vi "Transform And Project.vi"(11 "Scene in":refnum<class "Scene.lvclass">) -> (3 "Scene out":refnum<class "Scene.lvclass">)   [LabVIEW 2022 SP3, in "Application.lvlib" / "Scene.lvclass"]
uses:
  Scene.lvclass
  Libraries/3D/Vector 3D.ctl
  Scene.lvclass/Scene.ctl
  196e4586-e654-41ec-a3a4-43fea5068e8e.vi
  a59a4b44-279f-4314-be75-e28f6a03f0ec.vi
  <vilib>/Utility/High Resolution Relative Seconds.vi
  Libraries/3D/Normalise Vector.vi
  Libraries/3D/Multiply Vector By Matrix.vi
  Libraries/3D/Scale Point 3D (SGL) To Screen.vi
  Libraries/3D/Calculate Triangle Illumination.vi
  <vilib>/Utility/colorconv.llb/Color to RGB.vi
  Libraries/3D/Dot Product.vi
  <vilib>/Utility/colorconv.llb/RGB to Color.vi
  <userlib>/_OpenG.lib/array/array.llb/Sort Array__ogtk.vi
  <userlib>/_OpenG.lib/array/array.llb/Sort 1D Array (SGL)__ogtk.vi
  Libraries/3D/3D.lvlib
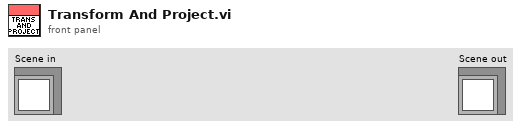
[diagram p1: front panel]
types:
  T1 = typedef "3D.lvlib/Vector 3D.ctl" = cluster{"x":sgl, "y":sgl, "z":sgl}
  T2 = typedef "3D.lvlib/Object.ctl" = cluster{"Triangles":T3[], "Diffuse Colour":u32, "Transform":T4}
  T3 = typedef "3D.lvlib/Triangle 3D.ctl" = cluster{"Point 1":T1, "Point 2":T1, "Point 3":T1}
  T4 = typedef "3D.lvlib/Transform.ctl" = cluster{"Position":T1, "Rotation":T1, "Scale":T1}
  T5 = typedef "Raster.lvlib/Screen Dimensions.ctl" = cluster{"Width":u32, "Height":u32}
  T6 = typedef "3D.lvlib/Triangle 3D With Colour.ctl" = cluster{"Point 1":T1, "Point 2":T1, "Point 3":T1, "Fill Colour":u32}
  T7 = typedef "3D.lvlib/Triangle 2D.ctl" = cluster{"Point 1":T8, "Point 2":T8, "Point 3":T8, "Fill Colour":u32}
  T8 = typedef "3D.lvlib/Point 2D.ctl" = cluster{"x":sgl, "y":sgl}
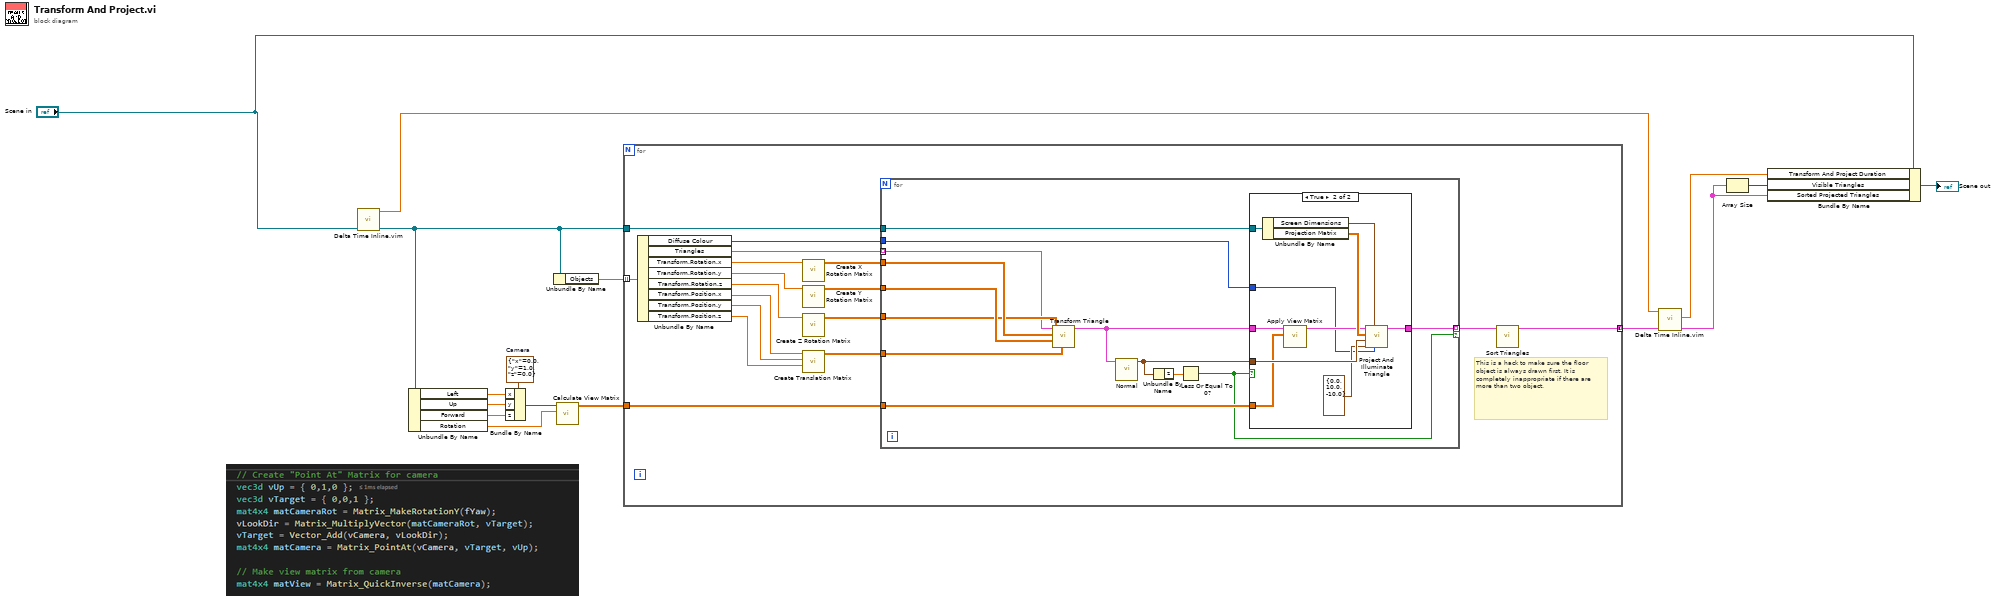
[diagram p0: block diagram]
diagram:
  w14 = T1 {"x"=0.0, "y"=1.0, "z"=0.0}  # Camera
  n1 = call "Delta Time Inline.vim"("value in"="Scene in") -> ("value out"=w16:refnum<class "Scene.lvclass">, "Relative Seconds out [s]"=w7:dbl)  [unwired: 8 in, 1 out]
  n2 = Unbundle By Name(w16) -> ("Left"=w9:sgl, "Up"=w10:sgl, "Forward"=w13:sgl, "Rotation"=w11:sgl)
  n3 = Bundle By Name(cluster=w14, "x"=w9, "y"=w10, "z"=w13) -> (w8:T1)
  n4 = Unbundle By Name(w16) -> ("Objects"=w15:T2[])
  n5 = call "Calculate View Matrix.vi"("Camera Rotation"=w11, "Camera Position"=w8) -> ("View Matrix"=w12:sgl[][])  [unwired: 9 in]
  n6 = for {
    tunnel: w16 -> [w33]
    tunnel: w15 -> [w26] mode=indexing
    tunnel: w12 -> [w27]
    tunnel: [w23] -> w6 mode=concatenating
    # "This is a hack to make sure the floor object is always drawn first. It is completely inappropriate if there are more than two object."
    n7 = Unbundle By Name(w26) -> ("Diffuse Colour"=w25:u32, "Triangles"=w32:T3[], "Transform.Rotation.x"=w22:sgl, "Transform.Rotation.y"=w21:sgl, "Transform.Rotation.z"=w20:sgl, "Transform.Position.x"=w19:sgl, "Transform.Position.y"=w18:sgl, "Transform.Position.z"=w17:sgl)
    n8 = call "Create X Rotation Matrix.vi"("Theta (°)"=w22) -> ("Rotation X Matrix"=w29:sgl[][])  [unwired: 10 in]
    n9 = call "Create Y Rotation Matrix.vi"("Theta (°)"=w21) -> ("Rotation Y Matrix"=w30:sgl[][])  [unwired: 10 in]
    n10 = call "Create Z Rotation Matrix.vi"("Theta (°)"=w20) -> ("Rotation Z Matrix"=w28:sgl[][])  [unwired: 10 in]
    n11 = call "Create Translation Matrix.vi"("z"=w17, "y"=w18, "x"=w19) -> ("Translation Matrix"=w31:sgl[][])  [unwired: 8 in]
    n12 = for {
      tunnel: w28 -> [w41]
      tunnel: w29 -> [w43]
      tunnel: [w45] -> w24 mode=indexing if=w36
      tunnel: w30 -> [w42]
      tunnel: w31 -> [w40]
      tunnel: w33 -> [w39]
      tunnel: w32 -> [w35] mode=indexing
      tunnel: w27 -> [w38]
      tunnel: w25 -> [w34]
      n13 = call "Transform Triangle.vi"("Translation Matrix"=w40, "Rotation Z Matrix"=w41, "Rotation Y Matrix"=w42, "Rotation X Matrix"=w43, "Triangle in"=w35) -> ("Triangle out"=w37:T3)  [unwired: 6 in]
      n14 = call "Normal.vi"("Triangle"=w37) -> ("Normal"=w44:T1)  [unwired: 10 in]
      n15 = Unbundle By Name(w44) -> ("z"=w46:sgl)
      n16 = Less Or Equal To 0?(x=w46) -> (x <= 0?=w36:bool)
      n17 = case shown="True" w36 {
        tunnel: [_ w56] -> w45
        tunnel: w44 -> [_ w52]
        tunnel: w39 -> [_ w55]
        tunnel: w37 -> [_ w50]
        tunnel: w38 -> [_ w49]
        tunnel: w34 -> [_ w47]
        frame False {
        }
        frame True {
          n18 = Unbundle By Name(w55) -> ("Screen Dimensions"=w54:T5, "Projection Matrix"=w53:sgl[][])
          n19 = call "Apply View Matrix.vi"("View Matrix"=w49, "Triangle in"=w50) -> ("Triangle"=w51:T3)  [unwired: 9 in]
          n20 = call "Project And Illuminate Triangle.vi"("Diffuse Colour"=w47, "Screen Dimensions"=w54, "Light Direction"=T1 {"x"=0.0, "y"=10.0, "z"=-10.0}, "Normal"=w52, "Projection Matrix"=w53, "Triangle in"=w51) -> ("Triangle"=w56:T6)  [unwired: 5 in]
        }
      }
    }
    n21 = call "Sort Triangles.vi"("Triangles"=w24) -> ("Triangles Sorted"=w23:T7[])  [unwired: 10 in]
  }
  n22 = call "Delta Time Inline.vim"("value in"=w6, "Relative Seconds in [s]"=w7) -> ("value out"=w3:T7[], "Delta Time [s]"=w2:dbl)  [unwired: 7 in, 1 out]
  n23 = Array Size(array=w3) -> (size(s)=w1:i32)
  n24 = Bundle By Name(cluster="Scene in", "Transform And Project Duration"=w2, "Visible Triangles"=w1, "Sorted Projected Triangles"=w3) -> (→"Scene out":refnum<class "Scene.lvclass">)
